vi "setup_lc_ys.vi"(0 "didian":string, 4 "shuoming":string, 7 "zc_luodi_num":string, 9 "yw":string, 10 "id":string) -> (2 "error":errorcluster caption="error out 2")   [LabVIEW 2017, in "Lib_code.lvlib"]
uses:
  Lib_code.lvlib
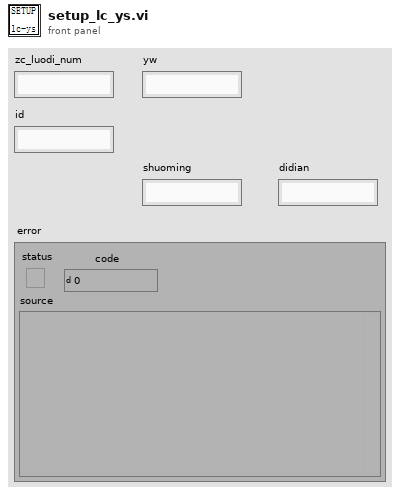
[diagram p1: front panel]
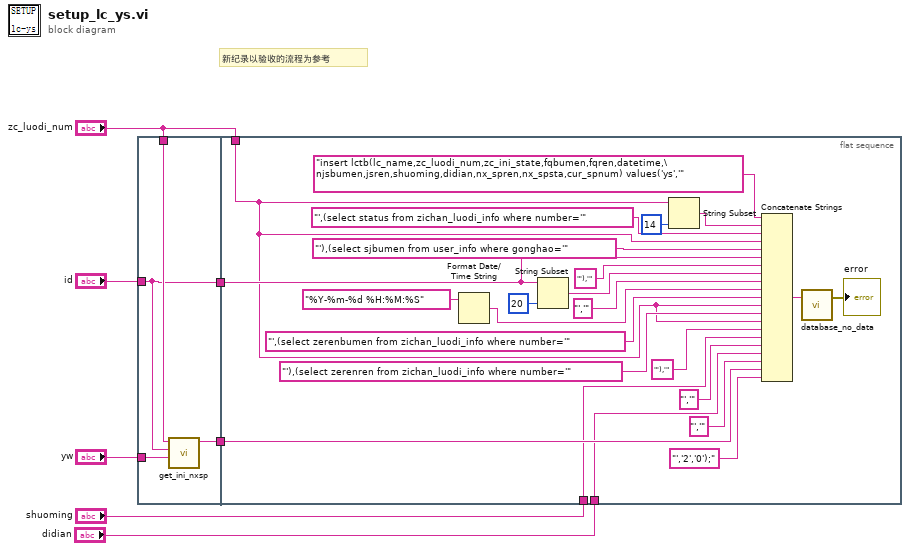
[diagram p0: block diagram]
diagram:
  # "新纪录以验收的流程为参考"
  n1 = flat-sequence {
    tunnel: "id" -> [w9]
    tunnel: [w9] -> w6
    tunnel: [w11] -> w5
    tunnel: "yw" -> [w8]
    tunnel: "zc_luodi_num" -> [w10]
    tunnel: w6 -> [w26]
    tunnel: w5 -> [w25]
    tunnel: "zc_luodi_num" -> [w12]
    tunnel: "shuoming" -> [w22]
    tunnel: "didian" -> [w17]
    frame #0 {
      n2 = call "get_ini_nxsp.vi"("yw"=w8, "id"=w9, "zc_luodi_num"=w10) -> ("sp_gonghao"=w11:string)  [unwired: 8 in]
    }
    frame #1 {
      n3 = Format Date/Time String(time format string (%c)="%Y-%m-%d %H:%M:%S" ("时间格式字符串(%c)")) -> (date/time string=w15:string)  [unwired: 2 in]
      n4 = String Subset(string=w26, length (rest)=20 ("长度（剩余）")) -> (substring=w28:string)  [unwired: 1 in]
      n5 = String Subset(string=w12, length (rest)=14 ("长度（剩余）")) -> (substring=w33:string)  [unwired: 1 in]
      n6 = Concatenate Strings("insert lctb(lc_name,zc_luodi_num,zc_ini_state,fqbumen,fqren,datetime,\njsbumen,jsren,shuoming,didian,nx_spren,nx_spsta,cur_spnum) values('ys','" ("格式字符串"), w33, "',(select status from zichan_luodi_info where number='" ("字符串"), w12, "'),(select sjbumen from user_info where gonghao='" ("字符串"), w26, "'),'" ("字符串"), w28, "','" ("字符串"), w15, "',(select zerenbumen from zichan_luodi_info where number='" ("字符串"), w12, "'),(select zerenren from zichan_luodi_info where number='" ("字符串"), w12, "'),'" ("字符串"), w22, "','" ("字符串"), w17, "','" ("字符串"), w25, "','2','0');" ("字符串")) -> (w20:string)
      n7 = call "database_no_data.vi"("input"=w20) -> ("error"=→"error":errorcluster)  [unwired: 2 in]
    }
  }
